vi "Status bar.vi"() -> (2 "Cancel Button 2":bool)   [LabVIEW 2014]
doc: "This VI shows the threshold value analysis is in process.\n\nDesigned by HB\nhaba@dtu.dk"
uses:
  Trigger Status Bar.vi
panel:
  out "Status":string
  in  "Cancel Button":bool
  in  "String":string="Performing threshold value analysis"
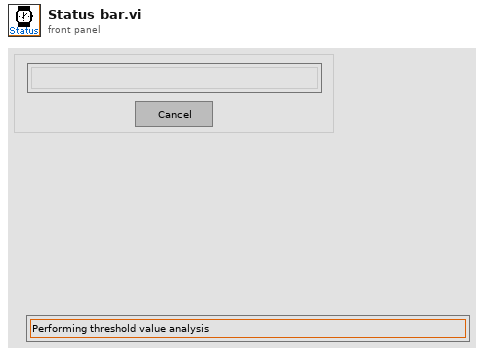
[diagram p1: front panel]
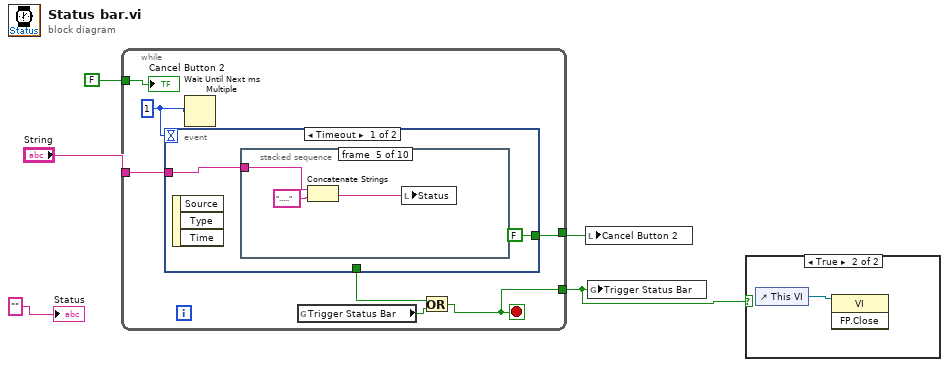
[diagram p0: block diagram]
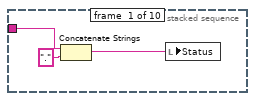
[diagram p3: hidden frame]
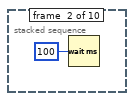
[diagram p4: hidden frame]
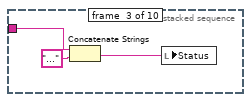
[diagram p5: hidden frame]
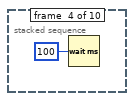
[diagram p6: hidden frame]
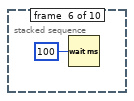
[diagram p7: hidden frame]
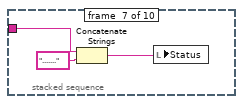
[diagram p8: hidden frame]
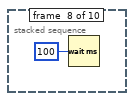
[diagram p9: hidden frame]
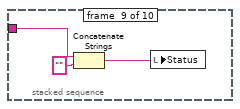
[diagram p10: hidden frame]
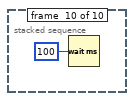
[diagram p11: hidden frame]
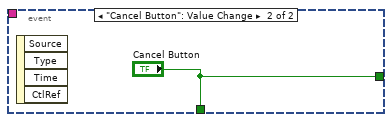
[diagram p12: hidden frame]
diagram:
  n1 = while {
    tunnel: "String" -> [w12]
    tunnel: [w10] -> w4
    tunnel: [w7] -> w1
    tunnel: FALSE ("Cancel Button 2") -> [w6]
    stop <- w10 stop-if-true
    w8 = 1
    n2 = event shown="[0] Timeout" {
      selector: _ -> [_ _]
      dyn-events: _ -> [_ _]
      timeout: w8 -> [_ _]
      tunnel: w12 -> [w14 _]
      tunnel: [_ "Cancel Button"] -> w9
      tunnel: [FALSE ("Cancel Button") "Cancel Button"] -> w7
      event Timeout {
        n3 = event-data() -> ()  [unwired: 1 in, 3 out]
        n4 = stacked-sequence {
          tunnel: w14 -> [w17 _ w19 _ w23 _ w27 _ w33 _]
          frame #0 {
            n5 = Concatenate Strings(w17, "." ("string")) -> (w15:string)
            n6 = local write "Status"(w15) -> ()
          }
          frame #1 {
            n7 = Wait (ms)(milliseconds to wait=u32 100) -> ()  [unwired: 1 out]
          }
          frame #2 {
            n8 = Concatenate Strings(w19, "..." ("string")) -> (w20:string)
            n9 = local write "Status"(w20) -> ()
          }
          frame #3 {
            n10 = Wait (ms)(milliseconds to wait=u32 100) -> ()  [unwired: 1 out]
          }
          frame #4 {
            n11 = Concatenate Strings(w23, "....." ("string")) -> (w24:string)
            n12 = local write "Status"(w24) -> ()
          }
          frame #5 {
            n13 = Wait (ms)(milliseconds to wait=u32 100) -> ()  [unwired: 1 out]
          }
          frame #6 {
            n14 = Concatenate Strings(w27, "......." ("string")) -> (w28:string)
            n15 = local write "Status"(w28) -> ()
          }
          frame #7 {
            n16 = Wait (ms)(milliseconds to wait=u32 100) -> ()  [unwired: 1 out]
          }
          frame #8 {
            n17 = Concatenate Strings(w33, "" ("string")) -> (w31:string)
            n18 = local write "Status"(w31) -> ()
          }
          frame #9 {
            n19 = Wait (ms)(milliseconds to wait=u32 100) -> ()  [unwired: 1 out]
          }
        }
      }
      event "Cancel Button": Value Change {
        n20 = event-data() -> ()  [unwired: 1 in, 4 out]
      }
    }
    n21 = Wait Until Next ms Multiple(millisecond multiple=w8) -> ()  [unwired: 1 out]
    n22 = global read "Trigger Status Bar.vi" "Trigger Status Bar"() -> (w11:bool)
    n23 = Or(x=w9, y=w11) -> (x .or. y?=w10:bool)
    "Cancel Button 2" <- w6
  }
  n24 = local write "Cancel Button 2"(w1) -> ()
  n25 = global write "Trigger Status Bar.vi" "Trigger Status Bar"(w4) -> ()
  n26 = case shown="True" w4 {
    frame False {
    }
    frame True {
      n27 = control-ref of="This VI"() -> (w36:refnum<vi>)
      n28 = invoke class="VI" method="FP.Close"(reference=w36) -> ()  [unwired: 2 in, 3 out]
    }
  }
  "Status" <- "" ("concatenated string")
